vi "Abort All numeric.vi"(11 "Test Case In":refnum<class "Tests Event MessengerM.lvclass">) -> (0 "error out":errorcluster, 3 "Test Case Out":refnum<class "Tests Event MessengerM.lvclass">)   [LabVIEW 2020, in "Tests Event MessengerM.lvclass"]
uses:
  Tests Event MessengerM.lvclass
  C:/Program Files/National Instruments/LabVIEW 2026/vi.lib/Astemes/LUnit/Test Case.lvclass
  <vilib>/Astemes/LUnit/Test Case.lvclass/Test Case.ctl
  <vilib>/Astemes/LUnit/Test Case.lvclass
  57c15532-2f4a-4f11-afcd-f221ee5c890e.vi
  f2c34a9e-f2e0-4be4-9fde-f0347f463bb0.vi
  7e5680cc-f493-4862-b9b2-60377483254e.vi
  fe735a7a-671a-40e2-ba6d-c493860db807.vi
  7cc3deff-b1cc-4ac5-8018-6614352e9d0d.vi
panel:
  out "msg":i32
  out "aborted? 2":bool
  out "aborted?":bool
  out "msg 2":i32
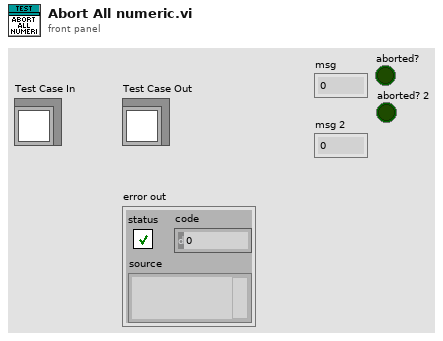
[diagram p1: front panel]
types:
  T1 = typedef "Event MessengerM-i32.lvlib/))Channel.ctl" = refnum<queue>
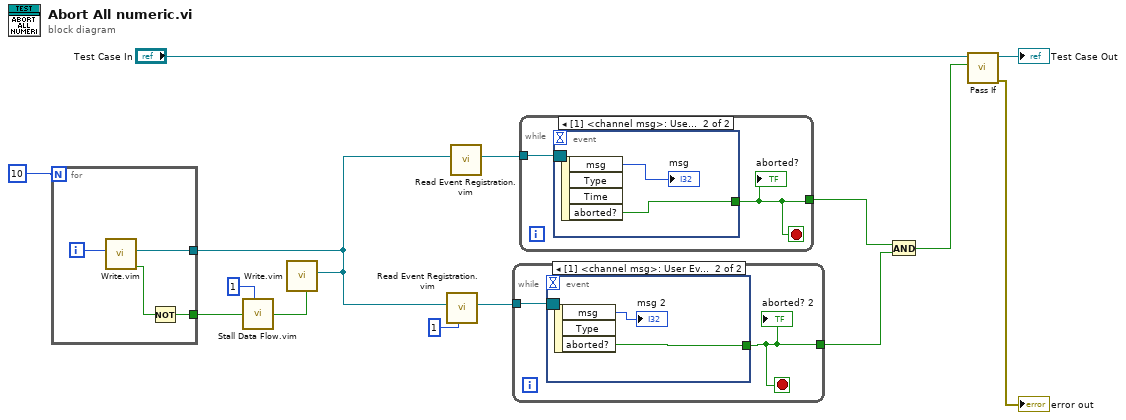
[diagram p0: block diagram]
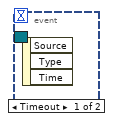
[diagram p2: hidden frame]
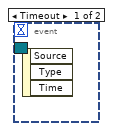
[diagram p3: hidden frame]
diagram:
  n1 = for {
    N: 10 -> [_]
    tunnel: [w18] -> w7
    tunnel: [w16] -> w2
    i -> [w17]
    n2 = call "Write.vim"("element"=w17) -> ("done?"=w15:bool, "channel"=w16:T1)  [unwired: 9 in]
    n3 = Not(x=w15) -> (.not. x?=w18:bool)
  }
  n4 = call "Stall Data Flow.vim"("value in"=w7, "milliseconds to wait"=u32 1) -> ("value out"=w1:bool)  [unwired: 1 out]
  n5 = call "Write.vim"("channel"=w2, "abort all (F)"=w1) -> ()  [unwired: 9 in, 1 out]
  n6 = call "Read Event Registration.vim"("subchannel"=1 ("subchannel (0)"), "channel"=w2) -> ("event registration refnum"=w5:refnum<event-registration>)  [unwired: 9 in]
  n7 = call "Read Event Registration.vim"("channel"=w2) -> ("event registration refnum"=w4:refnum<event-registration>)  [unwired: 10 in]
  n8 = while {
    tunnel: w5 -> [w20]
    tunnel: [w19] -> w9
    stop <- w19 stop-if-true
    n9 = event shown="[1] <channel msg>: User Event" {
      selector: w20 -> [_ _]
      dyn-events: _ -> [_ _]
      timeout: _ -> [_ _]
      tunnel: [_ w22] -> w19
      event Timeout {
        n10 = event-data() -> ()  [unwired: 1 in, 3 out]
      }
      event User Event {
        n11 = event-data() -> ("msg"=→"msg 2":i32, "aborted?"=w22:bool)  [unwired: 1 in, 1 out]
      }
    }
    "aborted? 2" <- w19
  }
  n12 = while {
    tunnel: w4 -> [w24]
    tunnel: [w23] -> w8
    stop <- w23 stop-if-true
    n13 = event shown="[1] <channel msg>: User Event" {
      selector: w24 -> [_ _]
      dyn-events: _ -> [_ _]
      timeout: _ -> [_ _]
      tunnel: [_ w26] -> w23
      event Timeout {
        n14 = event-data() -> ()  [unwired: 1 in, 3 out]
      }
      event User Event {
        n15 = event-data() -> ("msg"=→"msg":i32, "aborted?"=w26:bool)  [unwired: 1 in, 2 out]
      }
    }
    "aborted?" <- w23
  }
  n16 = And(x=w8, y=w9) -> (x .and. y?=w10:bool)
  n17 = call <vilib>:"Pass If.vi"("Pass?"=w10, "LUnit Test Case In"="Test Case In") -> ("error out"=→"error out":errorcluster, "LUnit Test Case Out"=→"Test Case Out":refnum<class "Tests Event MessengerM.lvclass">)  [unwired: 8 in]
